vi "checkPauseTimeElapsed.vi"(8 "error in (no error)":errorcluster, 11 "TestMonitor in":refnum<class "TestMonitor.lvclass">) -> (0 "error out":errorcluster, 2 "pauseTimeElapsedIsTrue":bool, 3 "TestMonitor out":refnum<class "TestMonitor.lvclass">)   [LabVIEW 2015]
uses:
  TestMonitor.lvclass
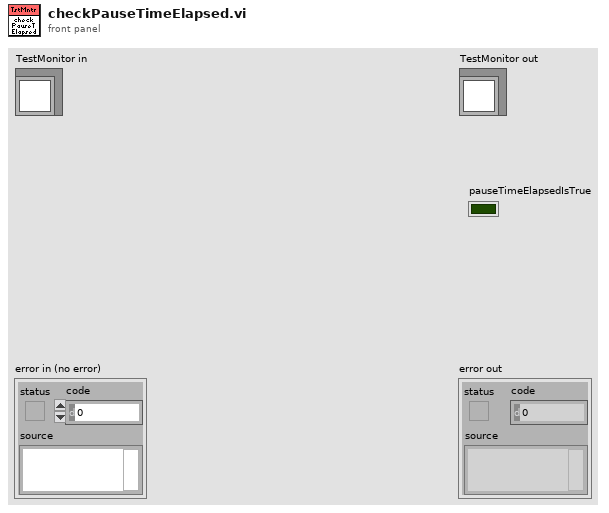
[diagram p1: front panel]
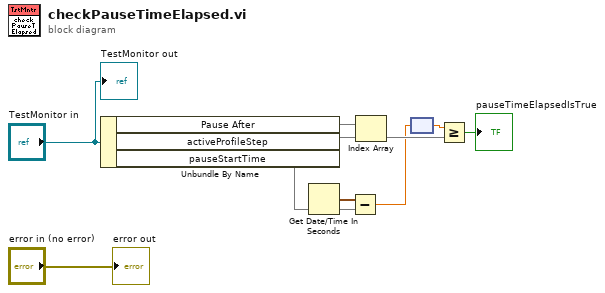
[diagram p0: block diagram]
diagram:
  n1 = Unbundle By Name("TestMonitor in") -> ("Pause After"=w6, "activeProfileStep"=w5, "pauseStartTime"=w7)
  n2 = Get Date/Time In Seconds() -> (seconds since 1Jan1904=w8:timestamp)
  n3 = Subtract(x=w8, y=w7) -> (x-y=w3:dbl)
  n4 = Index Array(array=w6, index=w5) -> (element=w4)
  n5 = node(w3) -> (w2:dbl[unit])
  n6 = Greater Or Equal?(x=w2, y=w4) -> (x >= y?=→"pauseTimeElapsedIsTrue":bool)
  "error out" <- "error in (no error)"
  "TestMonitor out" <- "TestMonitor in"
